vi "FPGA_8a_2ws_BIdireccional_Inycom.vi"() -> ()   [LabVIEW 2015]
uses:
  <vilib>/LabVIEW Targets/FPGA/cRIO/shared/nicrio_ModuleControls/nicrio_cRIO-9234_DataRatesRing2.ctl
  <vilib>/LabVIEW Targets/FPGA/cRIO/shared/nicrio_ModuleControls/nicrio_BasicConversionTime.ctl
  <vilib>/rvi/Emulation/niFpgaGetClockAttributes.vi
  <vilib>/rvi/Emulation/niFpgaSctlEmulationGetInTimedLoop.vi
  <vilib>/rvi/Emulation/niFpgaEmulationReportErrorSimple.vi
  <vilib>/rvi/Emulation/niFpgaProcessEmulError.vi
  <vilib>/rvi/eio/common/nirviEmuTemplateMethod_errors.vi
  <vilib>/rvi/Emulation/niFpgaCriticalErrorInLSC.vi
  <vilib>/rvi/eio/common/nirviEmuTemplatePropertySet_errors.vi
  <vilib>/rvi/interface/RandomDataEmulation/niFpgaRandomDataHandleErrors.vi
  <vilib>/eio/EIONode/EIONode.xnode
  <vilib>/eio/EIOPropertyNode/EIOPropertyNode.xnode
  <vilib>/rvi/DataTransferAndStorage/Container/XNode/niFpgaContainer.xnode
  <vilib>/rvi/interface/RandomDataEmulation/nirviRandomDataFpgaReadWriteTemplate.vi
  <vilib>/rvi/eio/common/nirviEmuTemplatePropertyGet_errors.vi
  <vilib>/rvi/eio/common/nirviEmuTemplatePropertyGet_noerrors.vi
  <vilib>/rvi/eio/common/nirviEmuTemplatePropertySet_noerrors.vi
panel:
  out "Numeric 2":i32
  out "WhlCnt1":fxp<+/-,24,-4> format="%.27g"
  in  "Offset_WS1":fxp<+/-,24,-4>=0.000999998301267624 format="%.27g"
  out "Rueda1?":i16
  out "WhlCnt2":fxp<+/-,24,-4> format="%.27g"
  out "Rueda2?":i16
  out "RuedaDetectada1?":bool
  out "RuedaDetectada2?":bool
  out "Parar":bool
  out "Nº Ruedas 1":i32
  out "NºRuedas 2":i32
  in  "Offset_WS2":fxp<+/-,24,-4>=0.000999998301267624 format="%.27g"
  in  "Cycles to Filter":u16=5
  in  "Canal cero WS1?":bool=TRUE
  in  "Canal cero WS2?":bool=TRUE
  in  "Conversion Time":T1
  in  "Count(mSec)":u32=2
  in  "Stop":bool
  out "Buffer Underflow":bool
  in  "Digital?":bool=TRUE
  out "medidas":fxp<+/-,24,4>[](array[numeric])
  out "Buffer Overflow":bool
  out "Error Out":errorcluster
  in  "Data Rate":T2=2 items=["51.200 kS/s (NI 9234)"=1, "25.600 kS/s (NI 9234)"=2, "17.067 kS/s (NI 9234)"=3, "12.800 kS/s (NI 9234)"=4, "10.240 kS/s (NI 9234)"=5, "8.533 kS/s (NI 9234)"=6, "7.314 kS/s (NI 9234)"=7, "6.400 kS/s (NI 9234)"=8, "5.689 kS/s (NI 9234)"=9, "5.120 kS/s (NI 9234)"=10, "4.654 kS/s (NI 9234)"=11, "4.267 kS/s (NI 9234)"=12, "3.938 kS/s (NI 9234)"=13, "3.657 kS/s (NI 9234)"=14, "3.413 kS/s (NI 9234)"=15, "3.200 kS/s (NI 9234)"=16, "3.012 kS/s (NI 9234)"=17, "2.845 kS/s (NI 9234)"=18, "2.695 kS/s (NI 9234)"=19, "2.560 kS/s (NI 9234)"=20, "2.438 kS/s (NI 9234)"=21, "2.328 kS/s (NI 9234)"=22, "2.226 kS/s (NI 9234)"=23, "2.133 kS/s (NI 9234)"=24, "2.048 kS/s (NI 9234)"=25, "1.969 kS/s (NI 9234)"=26, "1.896 kS/s (NI 9234)"=27, "1.829 kS/s (NI 9234)"=28, "1.765 kS/s (NI 9234)"=29, "1.707 kS/s (NI 9234)"=30, "1.652 kS/s (NI 9234)"=31]
  out "DC OK":bool
  in  "Fotocélula":bool
  out "Detector de\npresencia":bool
  out "Chassis Temperature":i16
  out "Direccion 0?":bool
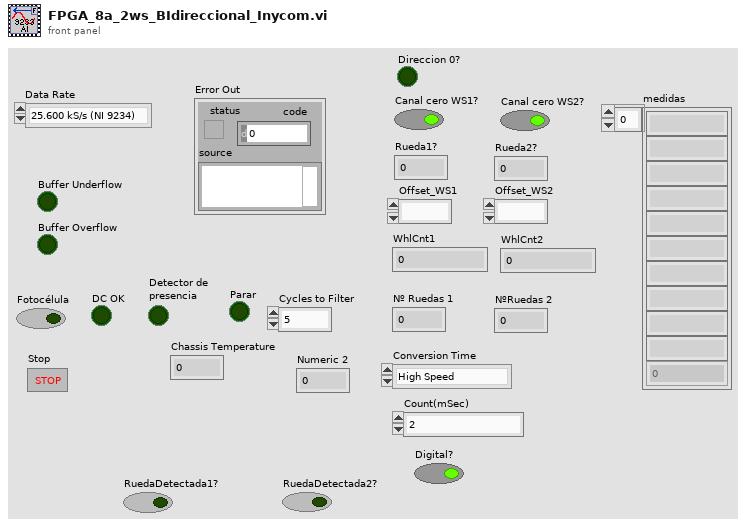
[diagram p1: front panel]
types:
  T1 = typedef "nicrio_BasicConversionTime.ctl" = enum8{"High Speed", "High Resolution"}
  T2 = typedef "nicrio_cRIO-9234_DataRatesRing2.ctl" = u8
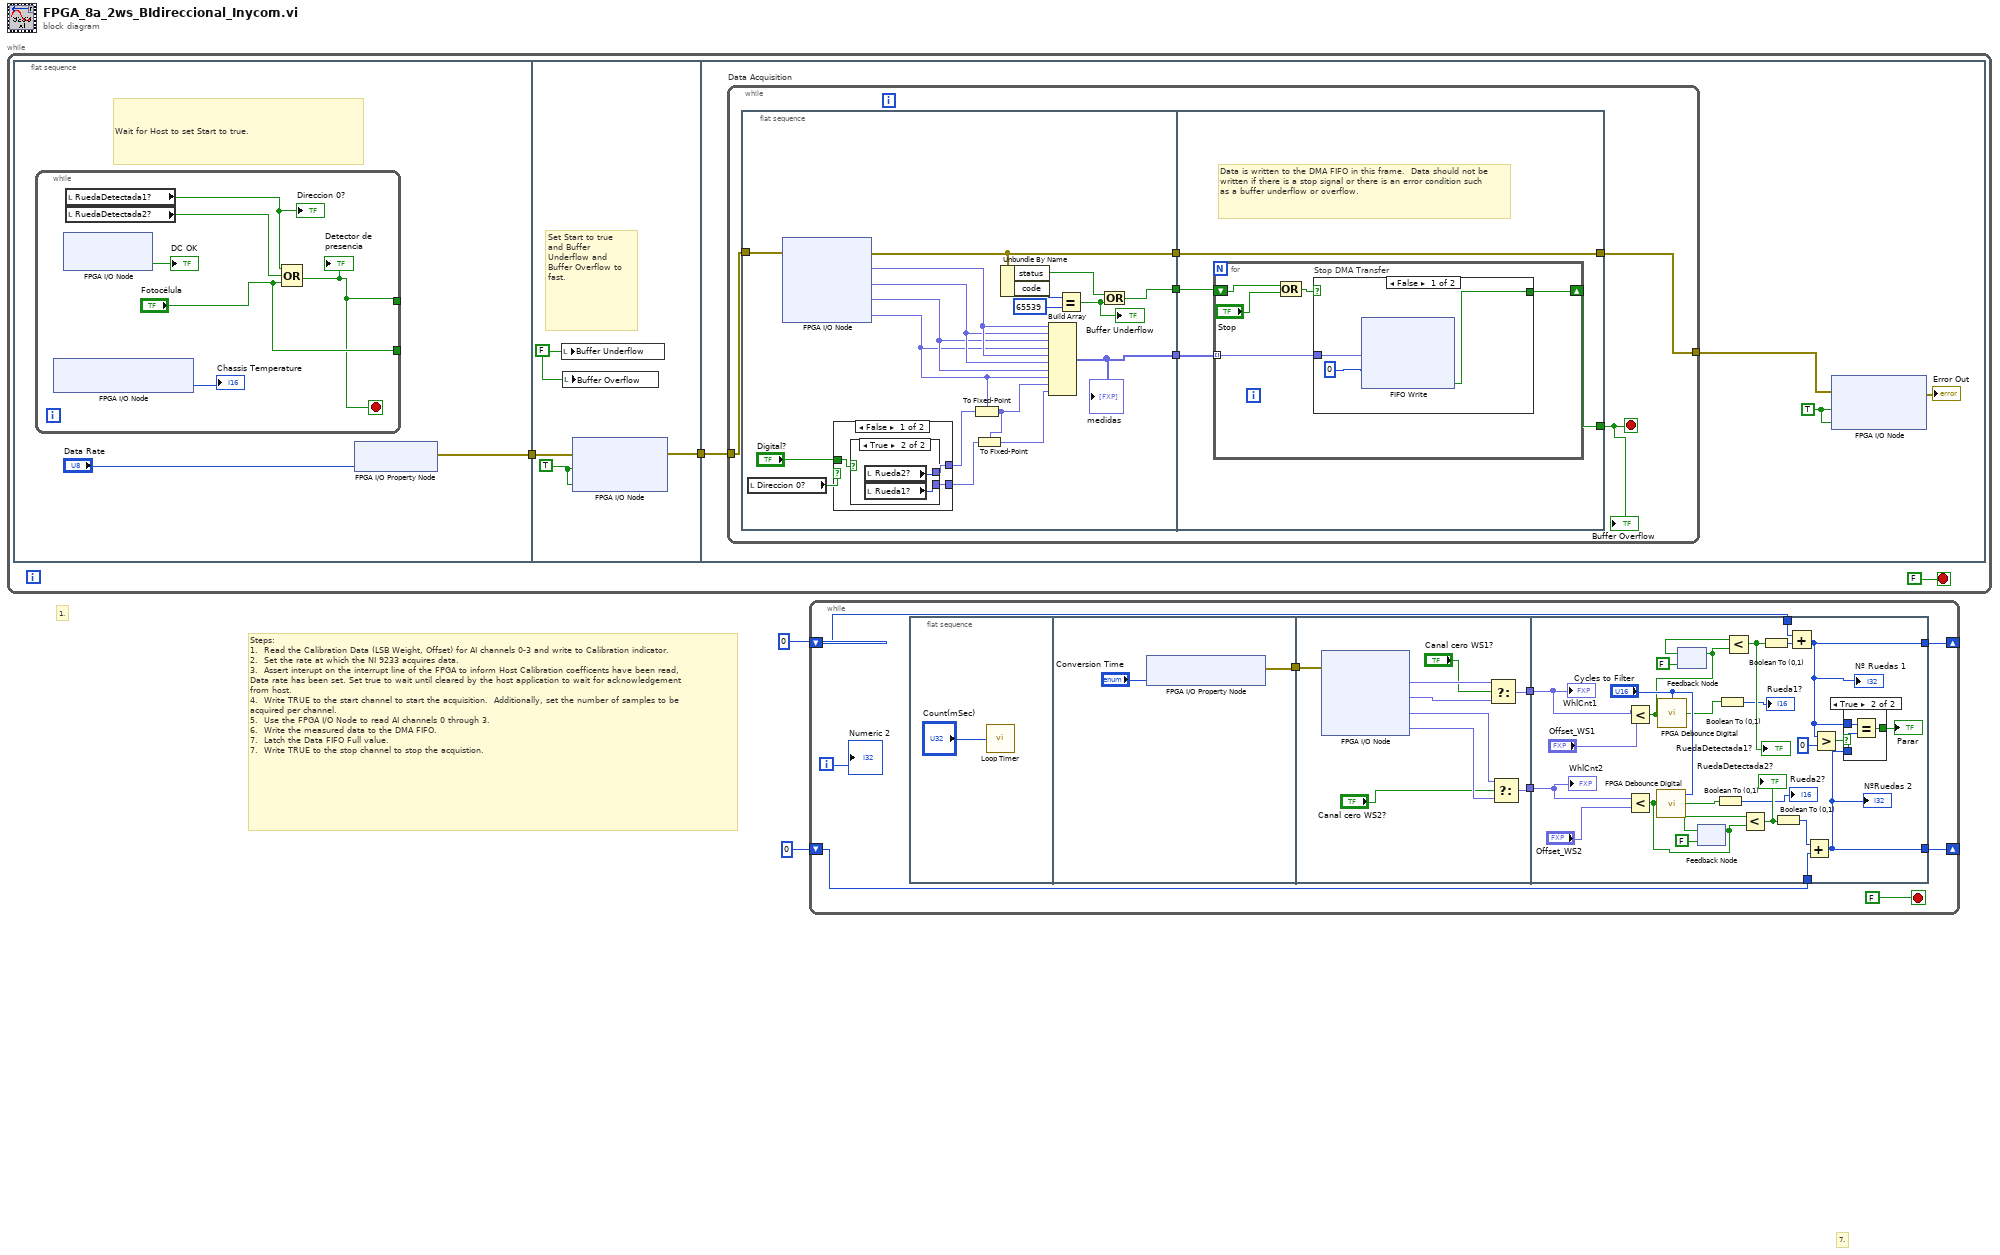
[diagram p0: block diagram]
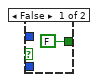
[diagram p2: hidden frame]
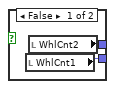
[diagram p3: hidden frame]
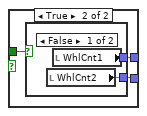
[diagram p4: hidden frame]
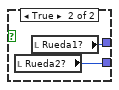
[diagram p5: hidden frame]
diagram:
  # "Steps: \n1.  Read the Calibration Data (LSB Weight, Offset) for AI channels 0-3 and write to Calibration indicator.\n2.  Set the rate at which the NI 9233 acquires data. \n3.  Assert interupt on the interrupt line of the FPGA to inform Host Calibration coefficents have been read, Data rate has been set. Set true to wait until cleared by the host application to wait for acknowledgement from host.\n4.  Write TRUE to the start channel to start the acquisition.  Additionally, set the number of samples to be acquired per channel.\n5.  Use the FPGA I/O Node to read AI channels 0 through 3. \n6.  Write the measured data to the DMA FIFO.\n7.  Latch the Data FIFO Full value.\n7.  Write TRUE to the stop channel to stop the acquistion."
  # "1."
  # "7."
  n1 = while {
    stop <- FALSE stop-if-true
    n2 = flat-sequence "MainSeq" {
      tunnel: [w7] -> w4
      tunnel: w4 -> [w16]
      tunnel: [w15] -> w3
      tunnel: w3 -> [w21]
      frame #0 {
        # "Wait for Host to set Start to true."
        n3 = while "initWait" {
          tunnel: ["Fotocélula"] -> _
          tunnel: [w9] -> _
          stop <- w9 stop-if-true
          n4 = xnode "FPGA I/O Node"() -> ("Chassis Temperature"=→"Chassis Temperature":i16)  [unwired: 1 in, 1 out]
          n5 = xnode "FPGA I/O Node"() -> ("Mod3/DI2"=→"DC OK":bool)  [unwired: 2 in, 2 out]
          n6 = local read "RuedaDetectada1?"() -> (w8:bool)
          "Direccion 0?" <- w8
          n7 = local read "RuedaDetectada2?"() -> (w10:bool)
          n8 = Compound Arithmetic op=OR(w8, w10, "Fotocélula") -> (w9:bool)
          "Detector de\npresencia" <- w9
        }
        n9 = xnode "FPGA I/O Property Node"("Data Rate"="Data Rate") -> ("error out"=w7:errorcluster)  [unwired: 2 in, 1 out]
      }
      frame #1 {
        w14 = TRUE
        w17 = FALSE ("Late? (Latched)")
        # "Set Start to true and Buffer Underflow and Buffer Overflow to fast."
        n10 = local write "Buffer Underflow"(w17) -> ()
        n11 = local write "Buffer Overflow"(w17) -> ()
        n12 = xnode "FPGA I/O Node"("error in"=w16, "Mod1/Start"=w14, "Mod2/Start"=w14) -> ("error out"=w15:errorcluster)  [unwired: 2 in, 2 out]
      }
      frame #2 {
        w18 = TRUE
        n13 = while "Data Acquisition" {
          tunnel: w21 -> [w25]
          tunnel: [w24] -> w19
          stop <- w22 stop-if-true
          n14 = flat-sequence "Data Acquisition Sequence" {
            tunnel: [w45] -> w27
            tunnel: [w39] -> w26
            tunnel: w25 -> [w44]
            tunnel: [w43] -> w23
            tunnel: w27 -> [w63]
            tunnel: w26 -> [w62]
            tunnel: [w61] -> w22
            tunnel: [w60] -> w24
            tunnel: w23 -> [w60]
            frame #0 {
              n15 = local read "Direccion 0?"() -> (w35:bool)
              n16 = xnode "FPGA I/O Node"("error in"=w44) -> ("error out"=w43:errorcluster, "Mod2/AI0"=w31:fxp<+/-,24,4>, "Mod2/AI1"=w30:fxp<+/-,24,4>, "Mod2/AI2"=w29:fxp<+/-,24,4>, "Mod2/AI3"=w28:fxp<+/-,24,4>)  [unwired: 4 in, 4 out]
              n17 = case shown="False" w35 {
                tunnel: "Digital?" -> [w48 w55]
                tunnel: [w47 w54] -> w37
                tunnel: [w46 w53] -> w34
                frame False {
                  n18 = case shown="True" w48 {
                    tunnel: [w50 w52] -> w47
                    tunnel: [w49 w51] -> w46
                    frame False {
                      n19 = local read "WhlCnt1"() -> (w49:fxp<+/-,24,-4>)
                      n20 = local read "WhlCnt2"() -> (w50:fxp<+/-,24,-4>)
                    }
                    frame True {
                      n21 = local read "Rueda2?"() -> (w52:i16)
                      n22 = local read "Rueda1?"() -> (w51:i16)
                    }
                  }
                }
                frame True {
                  n23 = case shown="False" w55 {
                    tunnel: [w57 w59] -> w54
                    tunnel: [w56 w58] -> w53
                    frame False {
                      n24 = local read "WhlCnt2"() -> (w56:fxp<+/-,24,-4>)
                      n25 = local read "WhlCnt1"() -> (w57:fxp<+/-,24,-4>)
                    }
                    frame True {
                      n26 = local read "Rueda2?"() -> (w58:i16)
                      n27 = local read "Rueda1?"() -> (w59:i16)
                    }
                  }
                }
              }
              n28 = To Fixed-Point(fixed-point type=w28, number=w37) -> (fixed-point=w33:fxp<+/-,24,4>)
              n29 = To Fixed-Point(fixed-point type=w33, number=w34) -> (fixed-point=w32:fxp<+/-,24,4>)
              n30 = Unbundle By Name(w43) -> ("status"=w38:bool, "code"=w42:i32)
              n31 = Build Array(w31, w30, w29, w28, w31, w30, w29, w28, w33, w32) -> (w45:fxp<+/-,24,4>[])
              "medidas" <- w45
              n32 = Equal?(x=w42, y=65539) -> (x = y?=w40:bool)
              "Buffer Underflow" <- w40
              n33 = Or(x=w38, y=w40) -> (x .or. y?=w39:bool)
            }
            frame #1 {
              # "Data is written to the DMA FIFO in this frame.  Data should not be written if there is a stop signal or there is an error condition such as a buffer underflow or overflow."
              n34 = for "DMAWriteLoop" {
                tunnel: w63 -> [w68] mode=indexing
                shift-right: [w67] -> w61
                shift-left: w62 -> [w66]
                n35 = Compound Arithmetic op=OR(w66, "Stop") -> (w65:bool)
                n36 = case "Stop DMA Transfer" shown="False" w65 {
                  selector: w65 -> [_ w72]
                  tunnel: w68 -> [w69 _]
                  tunnel: [w71 w72] -> w67
                  frame False {
                    n37 = xnode ("FIFO Write")("Element"=w69, "Timeout"=0) -> ("Timed Out?"=w71:bool)  [unwired: 1 in, 1 out]
                  }
                  frame True {
                  }
                }
              }
            }
          }
          "Buffer Overflow" <- w22
        }
        n38 = xnode "FPGA I/O Node"("error in"=w19, "Mod1/Stop"=w18, "Mod2/Stop"=w18) -> ("error out"=→"Error Out":errorcluster)  [unwired: 2 in, 2 out]
      }
    }
  }
  n39 = while {
    shift-right: [w78] -> _
    shift-left: 0 -> [w77]
    shift-right: [w75] -> _
    shift-left: 0 -> [w76]
    i -> [w74]
    stop <- FALSE stop-if-true
    n40 = flat-sequence {
      tunnel: [w83] -> w80
      tunnel: [w93] -> w81
      tunnel: w80 -> [w87]
      tunnel: [w90] -> w79
      tunnel: w81 -> [w119]
      tunnel: w79 -> [w117]
      tunnel: [w107] -> w78
      tunnel: w77 -> [w114]
      tunnel: w76 -> [w112]
      tunnel: [w106] -> w75
      frame #0 {
        n41 = call "Loop Timer"("Count(mSec)"="Count(mSec)") -> ()  [unwired: 1 out]
      }
      frame #1 {
        n42 = xnode "FPGA I/O Property Node"("Conversion Time"="Conversion Time") -> ("error out"=w83:errorcluster)  [unwired: 2 in, 1 out]
      }
      frame #2 {
        n43 = xnode "FPGA I/O Node"("error in"=w87) -> ("Mod4/AI0"=w92:fxp<+/-,24,-4>, "Mod4/AI1"=w91:fxp<+/-,24,-4>, "Mod4/AI2"=w89:fxp<+/-,24,-4>, "Mod4/AI3"=w88:fxp<+/-,24,-4>)  [unwired: 4 in, 5 out]
        n44 = Select(t=w92, s="Canal cero WS1?", f=w91) -> (s? t:f=w93:fxp<+/-,24,-4>)
        n45 = Select(t=w89, s="Canal cero WS2?", f=w88) -> (s? t:f=w90:fxp<+/-,24,-4>)
      }
      frame #3 {
        n46 = Less?(x=w119, y="Offset_WS1") -> (x < y?=w97:bool)
        n47 = Less?(x=w117, y="Offset_WS2") -> (x < y?=w95:bool)
        n48 = call "FPGA Debounce Digital.vi"("Input Signal"=w95, "Cycles to Filter"="Cycles to Filter") -> ("Output Filtered Signal"=w94:bool)
        n49 = call "FPGA Debounce Digital.vi"("Input Signal"=w97, "Cycles to Filter"="Cycles to Filter") -> ("Output Filtered Signal"=w96:bool)
        n50 = feedback-in #1(w97) -> ()
        n51 = feedback #1(FALSE) -> (w115:bool)
        n52 = feedback #2(FALSE) -> (w108:bool)
        n53 = feedback-in #2(w95) -> ()
        n54 = Boolean To (0,1)(Boolean=w94) -> (0, 1=→"Rueda2?":i16)
        n55 = Boolean To (0,1)(Boolean=w96) -> (0, 1=→"Rueda1?":i16)
        n56 = Less?(x=w115, y=w97) -> (x < y?=w103:bool)
        "RuedaDetectada1?" <- w103
        n57 = Less?(x=w108, y=w95) -> (x < y?=w102:bool)
        "RuedaDetectada2?" <- w102
        n58 = Boolean To (0,1)(Boolean=w103) -> (0, 1=w99:i16)
        n59 = Boolean To (0,1)(Boolean=w102) -> (0, 1=w104:i16)
        n60 = Add(x=w114, y=w99) -> (x+y=w107:i32)
        "Nº Ruedas 1" <- w107
        n61 = Add(x=w104, y=w112) -> (x+y=w106:i32)
        "NºRuedas 2" <- w106
        n62 = Greater?(x=w107, y=i64 0) -> (0:w109:bool)
        n63 = case shown="True" w109 {
          tunnel: w106 -> [_ w123]
          tunnel: w107 -> [_ w122]
          tunnel: [FALSE w121] -> w111
          frame False {
          }
          frame True {
            n64 = Equal?(x=w122, y=w123) -> (x = y?=w121:bool)
          }
        }
        "Parar" <- w111
        "WhlCnt1" <- w119
        "WhlCnt2" <- w117
      }
    }
    "Numeric 2" <- w74
  }
